vi "Enqueue.vi"(8 "error in (no error)":errorcluster, 9 "timeout in ms (-1)":i32=-1, 10 "Data to Enqueue":refnum<class "Data.lvclass">, 11 "Queue in":refnum<class "Queue.lvclass">) -> (0 "error out":errorcluster, 1 "timed out?":bool, 3 "Queue out":refnum<class "Queue.lvclass">)   [LabVIEW 2020, in "Data.lvlib" / "Queue.lvclass"]
doc: "Enqueue a Data element on the queue."
uses:
  Queue.lvclass
  Data.lvclass
  Queue.lvclass/Queue.ctl
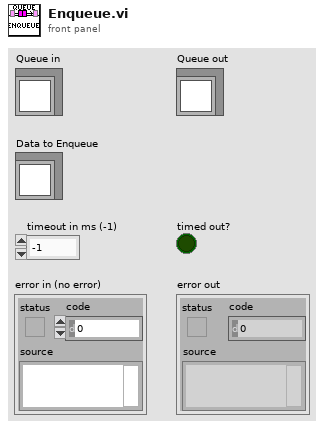
[diagram p1: front panel]
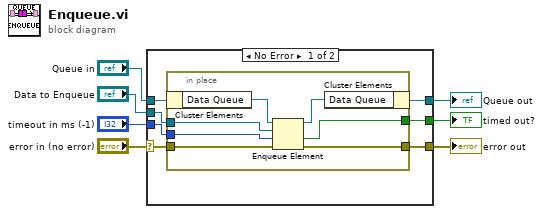
[diagram p0: block diagram]
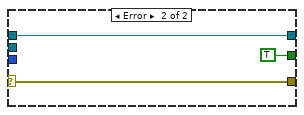
[diagram p2: hidden frame]
diagram:
  n1 = case shown="No Error" "error in (no error)" {
    selector: "error in (no error)" -> [w10 w24]
    tunnel: [w9 w24] -> w6
    tunnel: [w13 w23] -> w4
    tunnel: "Queue in" -> [w14 w23]
    tunnel: "Data to Enqueue" -> [w12 _]
    tunnel: "timeout in ms (-1)" -> [w11 _]
    tunnel: [w8 TRUE ("timed out?")] -> w1
    frame No Error {
      n2 = in-place {
        in-place-border: w12 -> [w19]
        in-place-border: w11 -> [w18]
        in-place-border: w10 -> [w17]
        in-place-border: [w16] -> w9
        in-place-border: [w15] -> w8
        n3 = in-place-cluster #1(w14) -> ("Data Queue"=w21:refnum<queue>)
        n4 = Enqueue Element(queue=w21, element=w19, timeout in ms (-1)=w18, error in (no error)=w17) -> (queue out=w20:refnum<queue>, timed out?=w15:bool, error out=w16:errorcluster)
        n5 = in-place-cluster #1("Data Queue"=w20) -> (w13:refnum<class "Queue.lvclass">)
      }
    }
    frame Error {
    }
  }
  "error out" <- w6
  "Queue out" <- w4
  "timed out?" <- w1
